vi "Smooth.vi"(2 "Y Input":dbl, 3 "X Input":dbl, 4 "Trigger":dbl) -> (0 "Y Output":dbl, 1 "X Output":dbl)   [LabVIEW 2016]
uses:
  <vilib>/Rock Robotics/Network Tables/NT Read Number.vi
  <vilib>/Rock Robotics/Network Tables/NT Read Boolean.vi
panel:
  in  "LowTrim":dbl=0.3
  in  "HighTrim":dbl=0.7
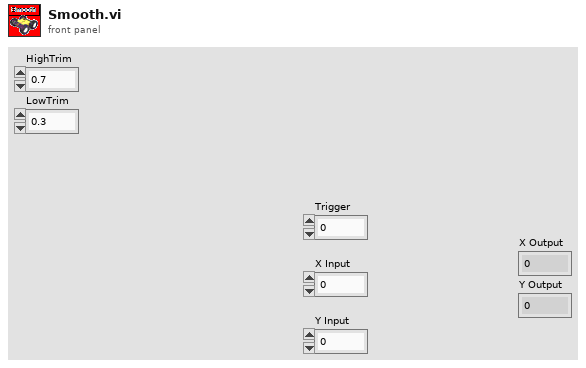
[diagram p1: front panel]
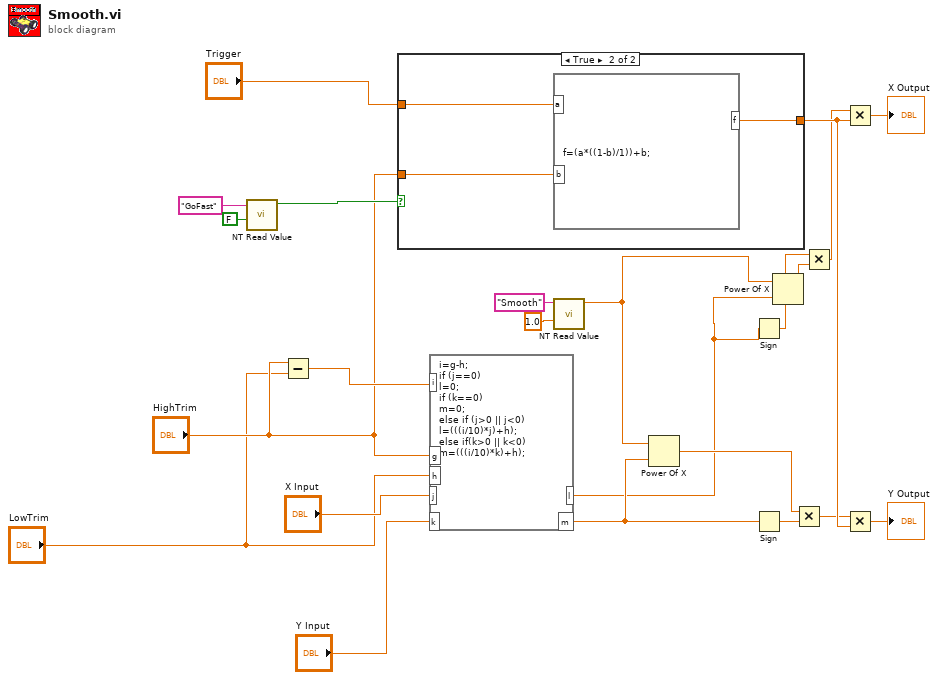
[diagram p0: block diagram]
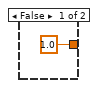
[diagram p2: hidden frame]
diagram:
  n1 = call-poly <vilib>:"NT Read Value.vi"("Default Value"=FALSE, "Name"="GoFast") -> ("Boolean"=w10:bool)  [unwired: 8 in, 1 out]
  n2 = Subtract(x="HighTrim", y="LowTrim") -> (x-y=w3:dbl)
  n3 = case shown="True" w10 {
    tunnel: [1.0 ("f") w25] -> w16
    tunnel: "HighTrim" -> [_ w26]
    tunnel: "Trigger" -> [_ w27]
    frame False {
    }
    frame True {
      n4 = formula code="f=(a*((1-b)/1))+b;"("a"=w27, "b"=w26) -> ("f"=w25:dbl)
    }
  }
  n5 = formula code="i=g-h;\nif (j==0)\nl=0;\nif (k==0)\nm=0;\nelse if (j>0 || j<0)\nl=(((i/10)*j)+h);\nelse if(k>0 || k<0)\nm=(((i/10)*k)+h);"("g"="HighTrim", "h"="LowTrim", "j"="X Input", "k"="Y Input", "i"=w3) -> ("l"=w5:dbl, "m"=w20:dbl)
  n6 = call-poly <vilib>:"NT Read Value.vi"("Default Value"=1.0, "Name"="Smooth") -> ("Numeric"=w22:dbl)  [unwired: 8 in, 1 out]
  n7 = Power Of X(1:w20, 2:w22) -> (0:w18:dbl)
  n8 = Sign(1:w5) -> (0:w4:dbl)
  n9 = Sign(1:w20) -> (0:w17:dbl)
  n10 = Power Of X(1:w5, 2:w22) -> (0:w19:dbl)
  n11 = Multiply(x=w18, y=w17) -> (x*y=w15:dbl)
  n12 = Multiply(x=w4, y=w19) -> (x*y=w14:dbl)
  n13 = Multiply(x=w14, y=w16) -> (x*y=→"X Output":dbl)
  n14 = Multiply(x=w15, y=w16) -> (x*y=→"Y Output":dbl)
